vi "Make_result_packet.vi"(2 "error in (no error)":errorcluster, 3 "Measuredata in":string[](array[string])) -> (0 "error out (no error)":errorcluster, 1 "String to Send":string)   [LabVIEW 2011]
doc: "Make_result_packet\n\nCreates a packet of all the results from the instruments to be sent to the client."
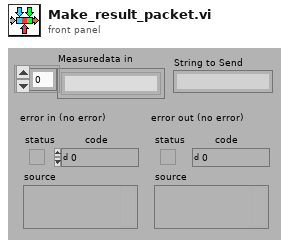
[diagram p1: front panel]
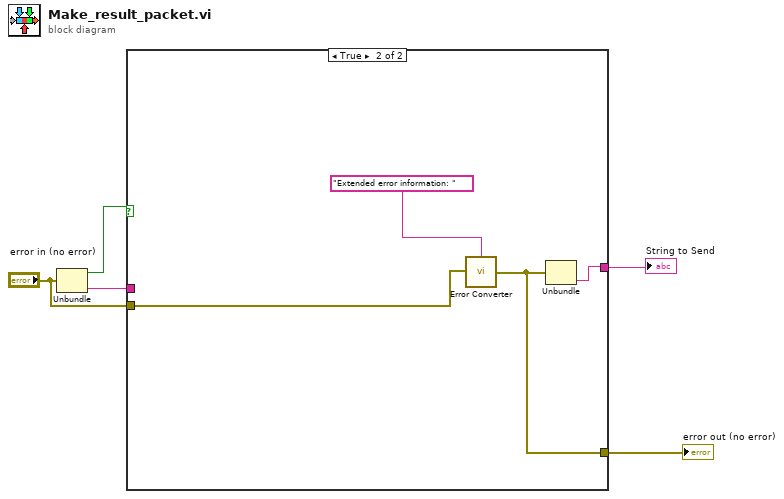
[diagram p0: block diagram]
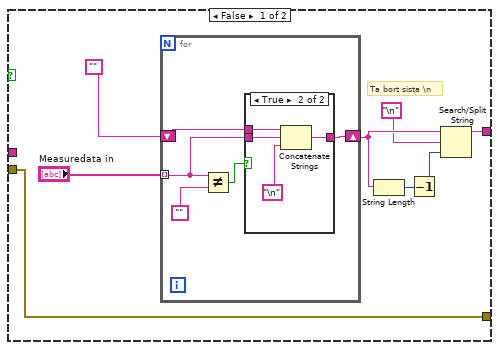
[diagram p2: hidden frame]
diagram:
  n1 = Unbundle("error in (no error)") -> ("status"=w5:bool, "source"=w3:string)  [unwired: 1 out]
  n2 = case shown="True" w5 {
    tunnel: [w7 w25] -> w4
    tunnel: w3 -> [_ _]
    tunnel: "error in (no error)" -> [w7 w26]
    tunnel: [w6 w24] -> w1
    frame False {
      # "Ta bort sista \\n"
      n3 = for {
        tunnel: "Measuredata in" -> [w15] mode=indexing
        shift-right: [w18] -> w10
        shift-left: "" -> [w17]
        n4 = Not Equal?(x=w15, y="") -> (x != y?=w16:bool)
        n5 = case shown="True" w16 {
          tunnel: [w19 w23] -> w18
          tunnel: w17 -> [w19 w22]
          tunnel: w15 -> [_ w20]
          frame False {
          }
          frame True {
            n6 = Concatenate Strings(w22, w20, "\n") -> (w23:string)
          }
        }
      }
      n7 = String Length(string=w10) -> (length=w11:i32)
      n8 = Decrement(x=w11) -> (x-1=w9:i32)
      n9 = Search/Split String(string=w10, search string/char (-)="\n", offset (0)=w9) -> (substring before match=w6:string)  [unwired: 2 out]
    }
    frame True {
      n10 = call "Error Converter.vi"("error in (no error)"=w26, "String to add to error message"="Extended error information: ") -> ("error out (no error)"=w25:errorcluster)
      n11 = Unbundle(w25) -> ("source"=w24:string)  [unwired: 2 out]
    }
  }
  "error out (no error)" <- w4
  "String to Send" <- w1
